vi "修改密码.vi"(9 "新密码":string, 10 "用户名":string, 11 "connection reference":T1) -> (0 "error out":errorcluster)   [LabVIEW 2013, in "数据库操作.lvclass"]
uses:
  <vilib>/addons/database/Connection.llb/Conn ObjectReference.ctl
  <vilib>/addons/database/Connection.llb/Conn Execute.vi
  <vilib>/addons/database/NI_Database_API.lvlib
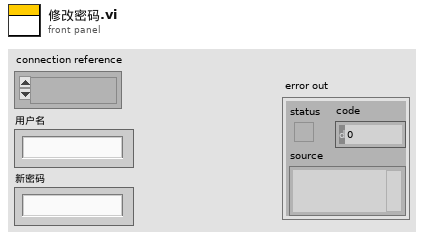
[diagram p1: front panel]
types:
  T1 = typedef "NI_Database_API.lvlib/Conn ObjectReference.ctl" = refnum<k1>
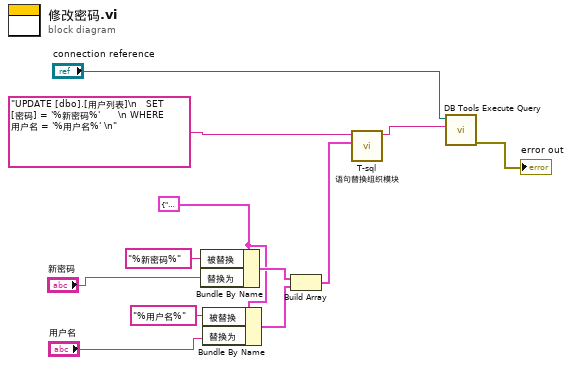
[diagram p0: block diagram]
diagram:
  w9 = cluster{"被替换":string, "替换为":string} {"被替换"="", "替换为"=""} ("替换单元")
  n1 = Bundle By Name(cluster=w9, "被替换"="%新密码%", "替换为"="新密码") -> (w10:cluster{"被替换":string, "替换为":string})
  n2 = Bundle By Name(cluster=w9, "被替换"="%用户名%", "替换为"="用户名") -> (w8:cluster{"被替换":string, "替换为":string})
  n3 = Build Array(w10, w8) -> (w7:cluster{"被替换":string, "替换为":string}[])
  n4 = call "T-sql 语句替换组织模块.vi"("替换项"=w7, "T-sql 模板"="UPDATE [dbo].[用户列表]\n   SET [密码] = '%新密码%'      \n WHERE 用户名 = '%用户名%' \n") -> ("T-sql"=w2:string)  [unwired: 8 in, 1 out]
  n5 = call-poly <vilib>:"DB Tools Execute Query.vi"("SQL query"=w2, "connection reference"="connection reference") -> ("error out"=→"error out":errorcluster)  [unwired: 6 in, 1 out]
